vi "A.vi"(1 "Y":dbl) -> (0 "A":dbl)   [LabVIEW 2012]
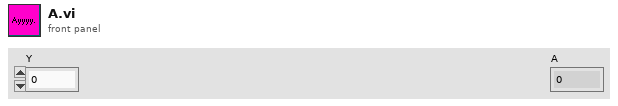
[diagram p1: front panel]
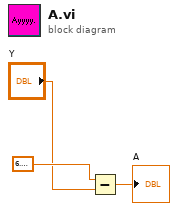
[diagram p0: block diagram]
diagram:
  n1 = Subtract(x=6.283185307179586, y="Y") -> (x-y=→"A":dbl)
